vi "hari seminar workout.vi"() -> ()   [LabVIEW 2020]
panel:
  out "Array 3":i32[](array[numeric])
  in  "Boolean":bool
  out "Array 2":i32[](array[numeric])
  out "Array":i32[](array[numeric])
  out "Numeric":i32
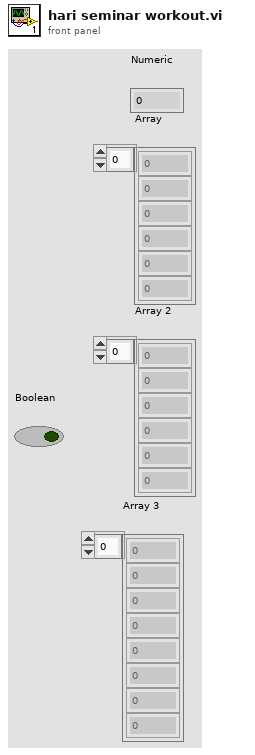
[diagram p1: front panel]
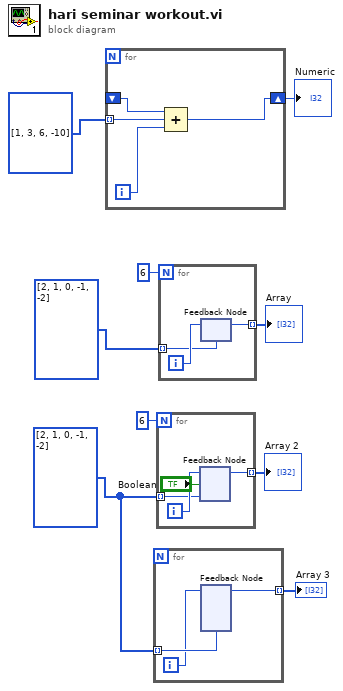
[diagram p0: block diagram]
diagram:
  w2 = i32[] [2, 1, 0, -1, -2]
  n1 = for {
    tunnel: i32[] [1, 3, 6, -10] -> [w13] mode=indexing
    shift-right: [w12] -> w9
    shift-left: _ -> [w10]
    i -> [w11]
    n2 = Compound Arithmetic op=ADD(w10, w13, w11) -> (w12:i32)
  }
  "Numeric" <- w9
  n3 = for {
    tunnel: w2 -> [w16] mode=indexing
    tunnel: [w14] -> w1 mode=indexing
    i -> [w15]
    n4 = feedback #1(w16) -> (w14:i32)
    n5 = feedback-in #1(w15) -> ()
  }
  "Array 3" <- w1
  n6 = for {
    N: 6 -> [_]
    tunnel: [w19] -> w3 mode=indexing
    tunnel: w2 -> [w18] mode=indexing
    i -> [w20]
    n7 = feedback #2(w18) -> (w19:i32)
    n8 = feedback-in #2(w20, "Boolean") -> ()
  }
  "Array 2" <- w3
  n9 = for {
    N: 6 -> [_]
    tunnel: [w22] -> w8 mode=indexing
    tunnel: i32[] [2, 1, 0, -1, -2] -> [w21] mode=indexing
    i -> [w23]
    n10 = feedback #3(w21) -> (w22:i32)
    n11 = feedback-in #3(w23) -> ()
  }
  "Array" <- w8
